vi "Periodicity.vi"() -> ()   [LabVIEW 2020]
uses:
  <vilib>/measure/NI_MABase.lvlib
  <vilib>/gmath/NI_Gmath.lvlib
panel:
  out "Period":dbl=2.0
  out "Fundamental Frequency":dbl=0.5
  out "Period":dbl[](array[numeric])=[1.0, 0.5, 0.4, 0.3333333333333333]
  in  "Stop":bool
  out "Summed Signals":waveform(dbl)(graph)={"t0"=timestamp(0 s since 1904-01-01), "dt"=0.01, "Y"=array[1000 elements]}
  out "Signals":waveform(dbl)[](graph)=[{"t0"=timestamp(0 s since 1904-01-01), "dt"=0.01, "Y"=array[1000 elements]}, {"t0"=timestamp(0 s since 1904-01-01), "dt"=0.01, "Y"=array[1000 elements]}, {"t0"=timestamp(0 s since 1904-01-01), "dt"=0.01, "Y"=array[1000 elements]}, {"t0"=timestamp(0 s since 1904-01-01), "dt"=0.01, "Y"=array[1000 elements]}]
  in  "Amplitude":dbl[](array[numeric])=[2.0, 1.0, 0.5, 1.0]
  in  "Phase [Deg]":dbl[](array[numeric])=[0.0, 90.0, 90.0, 0.0]
  in  "Frequency":dbl[](array[numeric])=[1.0, 2.0, 2.5, 3.0]
  # "Illustration of Periodic Signals"
  # "Add sine-waves of different frequency,\namplitude, and phase.\nPlot the resulting summed signal, and \nfind its periodicity."
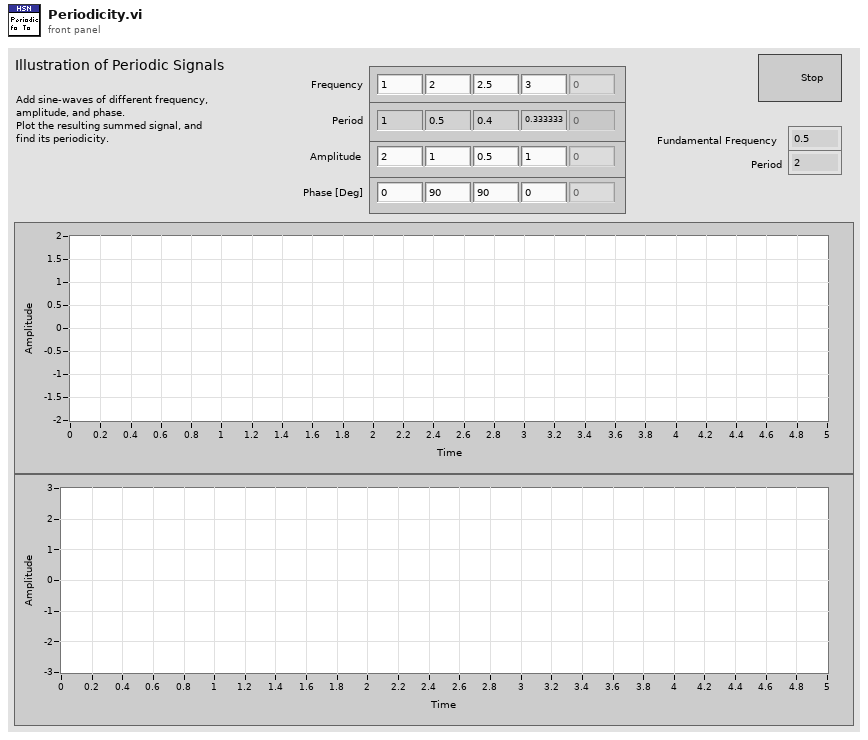
[diagram p1: front panel]
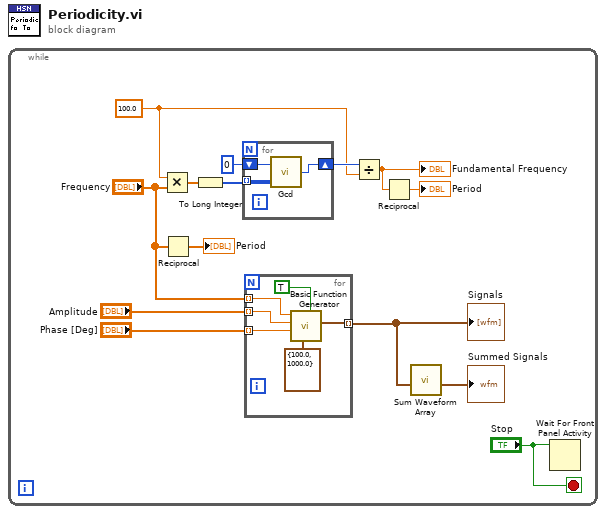
[diagram p0: block diagram]
diagram:
  n1 = while {
    stop <- "Stop" stop-if-true
    w5 = 100.0
    n2 = Multiply(x=w5, y="Frequency") -> (x*y=w8:dbl[])
    n3 = Reciprocal(x="Frequency") -> (1/x=→"Period":dbl[])
    n4 = To Long Integer(number=w8) -> (32bit integer=w7:i32[])
    n5 = for {
      tunnel: w7 -> [w17] mode=indexing
      shift-right: [w15] -> w6
      shift-left: 0 ("gcd(x,y)") -> [w16]
      n6 = call <vilib>:"Gcd.vi"("y"=w17, "x"=w16) -> ("gcd(x,y)"=w15:i32)
    }
    n7 = for {
      tunnel: "Frequency" -> [w23] mode=indexing
      tunnel: "Amplitude" -> [w22] mode=indexing
      tunnel: "Phase [Deg]" -> [w21] mode=indexing
      tunnel: [w19] -> w2 mode=indexing
      n8 = call <vilib>:"Basic Function Generator.vi"("reset signal"=TRUE, "sampling info"=cluster{"Fs":dbl, "#s":dbl} {"Fs"=100.0, "#s"=1000.0}, "phase"=w21, "amplitude"=w22, "frequency"=w23) -> ("signal out"=w19:waveform(dbl))  [unwired: 4 in, 2 out]
    }
    "Signals" <- w2
    n9 = Divide(x=w6, y=w5) -> (x/y=w4:dbl)
    "Fundamental Frequency" <- w4
    n10 = Reciprocal(x=w4) -> (1/x=→"Period":dbl)
    n11 = call "Sum Waveform Array.vi"("Waveform Array"=w2) -> ("Summed Waveform Array"=→"Summed Signals":waveform(dbl))  [unwired: 9 in, 1 out]
    n12 = Wait For Front Panel Activity(3:"Stop") -> ()  [unwired: 2 in, 1 out]
  }
